vi "Check Protection.vi"(8 "error in (no error)":errorcluster, 10 "String in":string, 11 "Checksum U8 in":refnum<class "Checksum U8.lvclass">) -> (0 "error out":errorcluster, 1 "Protection Error":errorcluster, 2 "String out":string, 3 "Checksum U8 out":refnum<class "Checksum U8.lvclass">)   [LabVIEW 2020, in "Protections.lvlib" / "Checksum U8.lvclass"]
uses:
  Checksum U8.lvclass
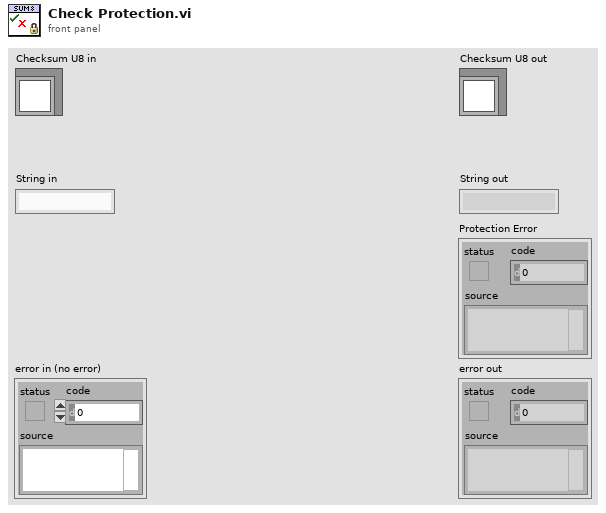
[diagram p1: front panel]
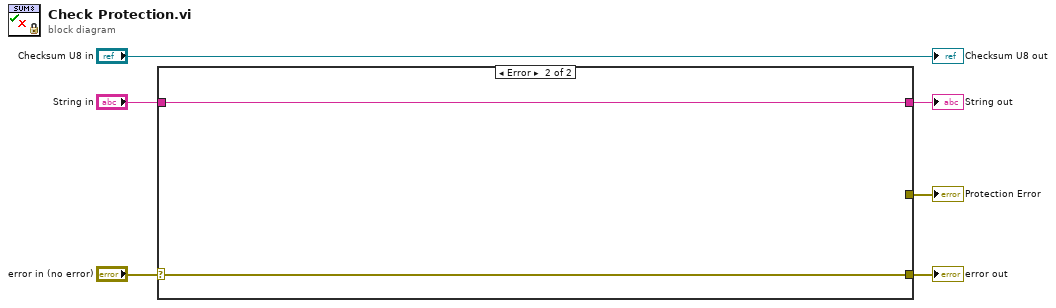
[diagram p0: block diagram]
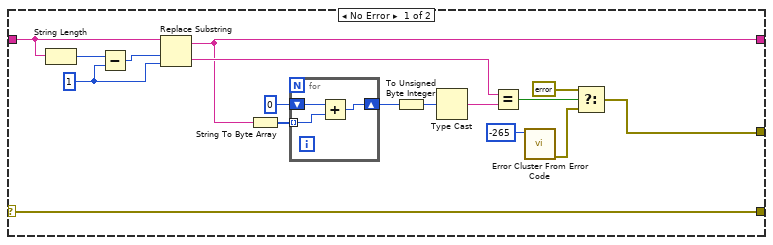
[diagram p2: hidden frame]
diagram:
  n1 = case shown="Error" "error in (no error)" {
    selector: "error in (no error)" -> [w7 w27]
    tunnel: "String in" -> [w11 w28]
    tunnel: [w9 _] -> w2
    tunnel: [w10 w28] -> w4
    tunnel: [w7 w27] -> w1
    frame No Error {
      w18 = 1
      n2 = String Length(string=w11) -> (length=w20:i32)
      n3 = Subtract(x=w20, y=w18) -> (x-y=w19:i32)
      n4 = Replace Substring(2:w18, 3:w19, 5:w11) -> (0:w16:string, 1:w10:string)  [unwired: 1 in]
      n5 = String To Byte Array(string=w10) -> (unsigned byte array=w23:u8[])
      n6 = for {
        tunnel: w23 -> [w26] mode=indexing
        shift-right: [w24] -> w21
        shift-left: u64 0 -> [w25]
        n7 = Add(x=w25, y=w26) -> (x+y=w24:u64)
      }
      n8 = To Unsigned Byte Integer(number=w21) -> (unsigned 8bit integer=w8:u8)
      n9 = Type Cast(x=w8) -> (*(type *) &x=w17:string)  [unwired: 1 in]
      n10 = Equal?(x=w16, y=w17) -> (x = y?=w15:bool)
      n11 = call <vilib>:"Error Cluster From Error Code.vi"("error code (0)"=-265) -> ("error out"=w13:errorcluster)  [unwired: 8 in]
      n12 = Select(t=errorcluster {"status"=FALSE, "code"=0, "source"=""} ("error in (no error)"), s=w15, f=w13) -> (s? t:f=w9:errorcluster)
    }
    frame Error {
    }
  }
  "error out" <- w1
  "String out" <- w4
  "Protection Error" <- w2
  "Checksum U8 out" <- "Checksum U8 in"
